vi "String Index Of From Test.vi"() -> ()   [LabVIEW 2014, in "ESP8266 WiFi Wrapper.lvlib"]
uses:
  <vilib>/Aledyne-TSXperts/Arduino Compatible Compiler for LabVIEW/addons/ESP8266 WiFi Wrapper/ESP8266 WiFi Wrapper.lvlib
panel:
  out "index":i8
  out "Error Out":errorcluster
  in  "Error In":errorcluster
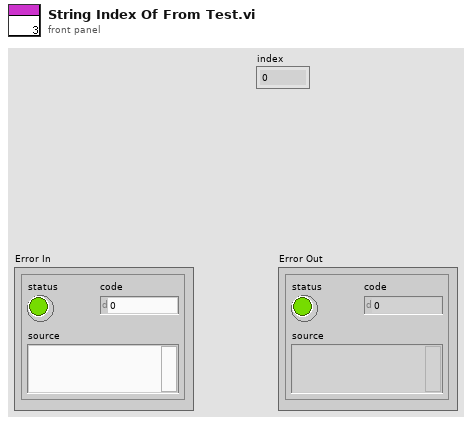
[diagram p1: front panel]
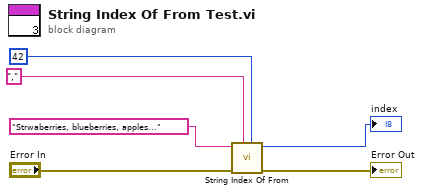
[diagram p0: block diagram]
diagram:
  n1 = call <vilib>:"String Index Of From.vi"("Start from"=u8 42, "Find string"=",", "Error In"="Error In", "Input String"="Strwaberries, blueberries, apples...") -> ("Error Out"=→"Error Out":errorcluster, "index"=→"index":i8)  [unwired: 6 in]
